vi "Digital_Bridge_3_kart.vi"() -> ()   [LabVIEW 2014] (continued)
                      n2699 = case shown="6" w6200 {
                        tunnel: [4.0 ("iterasyon WAGNER") w6203 w6204 w6205 w6206 w6207 w6208] -> w6199
                        frame 0, Default {
                        }
                        frame 1 {
                          n2700 = local read "Iterasyon Successful"() -> (w6203:dbl)
                        }
                        frame 2 {
                          n2701 = local read "Direnc 1 - Direnc 2"() -> (w6204:u32)
                        }
                        frame 3 {
                          n2702 = local read "olcum"() -> (w6205:u16)
                        }
                        frame 4 {
                          n2703 = local read "set"() -> (w6206:u16)
                        }
                        frame 5 {
                          n2704 = local read "frekans index"() -> (w6207:dbl)
                        }
                        frame 6 {
                          n2705 = local read "iterasyon WAGNER"() -> (w6208:dbl)
                        }
                      }
                      n2706 = Replace Array Subset(array=w6201, new element=w6199, index=w6200) -> (w6198:dbl[])
                    }
                    n2707 = local read "Output Denge Kosulu x2_y2"() -> (w6169:dbl[][])
                    n2708 = control-ref of="Default Values Listbox"() -> (w6148:refnum<vi>)
                    n2709 = local read "Output Denge Kosulu x1_x2"() -> (w6142:dbl[][])
                    n2710 = local read "Outpu Denge Kosulu y1_y2"() -> (w6143:dbl[][])
                    n2711 = local read "Cluster"() -> (w6146:T2)
                    n2712 = local read "Cluster 2"() -> (w6145:T1)
                    n2713 = local read "Frekanslar"() -> (w6129:dbl[])
                    n2714 = Array Size(array=w6129) -> (size(s)=w6128:i32)
                    n2715 = local read "default values"() -> (w6168:T3)
                    n2716 = local read "input values"() -> (w6147:dbl[])
                    n2717 = call "merge_x_y.vi"("frekans size"=w6128, "y1_y2"=w6143, "x1_x2"=w6142) -> ("x1_x2_y1_y2"=w6141:dbl[][])  [unwired: 8 in]
                    n2718 = local read "Sheet name"() -> (w6165:string)
                    n2719 = local read "Other Boolean Array"() -> (w6163:bool[])
                    n2720 = for {
                      N: 5 -> [_]
                      shift-right: [w6189] -> w6166
                      shift-left: w6163 -> [w6192]
                      i -> [w6191]
                      n2721 = case shown="0, Default" w6191 {
                        tunnel: [FALSE FALSE FALSE FALSE FALSE] -> w6190
                        frame 0, Default {
                        }
                        frame 1 {
                        }
                        frame 2 {
                        }
                        frame 3 {
                        }
                        frame 4 {
                        }
                      }
                      n2722 = Replace Array Subset(array=w6192, new element=w6190, index=w6191) -> (w6189:bool[])
                    }
                    n2723 = call "Pass.vi"("Other Array"=w6167, "Other Boolean Array"=w6166, "Denge Kosulu x2_y2"=w6169, "LstBox Refnum"=w6148, "Cluster"=w6146, "F/P Array Cluster"=w6145, "Sheet name"=w6165, "default values"=w6168, "x1_x2_y1_y2"=w6141, "input values"=w6147) -> ("output values"=w6140:dbl[], "Output Other Boolean Array"=w6161:bool[], "Output Cluster"=w6139:T2, "Output F/P Array Cluster"=w6135:T1, "output default values"=w6144:T11, "Output Iterasyon Successful"=w6162:dbl, "Denge Seçimi"=w6150:u8, "end time"=w6149:string)  [unwired: 1 in, 1 out]
                    n2724 = Unbundle By Name(w6139) -> ("F Values Array"=w6138:dbl[][], "control hz array"=w6137:dbl[][], "extra default values"=w6136:dbl[][])
                    n2725 = local write "input values"(w6140) -> ()
                    n2726 = Unbundle By Name(w6135) -> ("AD F/P Array"=w6134:dbl[][], "10R F/P Array"=w6133:dbl[][], "1R F/P Array"=w6132:dbl[][], "Wagner F/P Array"=w6131:dbl[][], "Kelvin F/P Array"=w6130:dbl[][])
                    n2727 = local write "default values"(w6144) -> ()
                    n2728 = local write "Iterasyon Successful"(w6162) -> ()
                    n2729 = local write "F Values Array"(w6138) -> ()
                    n2730 = local write "control hz array"(w6137) -> ()
                    n2731 = local write "extra default values"(w6136) -> ()
                    n2732 = local write "AD F/P Array"(w6134) -> ()
                    n2733 = local write "10R F/P Array"(w6133) -> ()
                    n2734 = local write "1R F/P Array"(w6132) -> ()
                    n2735 = local write "Wagner F/P Array"(w6131) -> ()
                    n2736 = local write "Kelvin F/P Array"(w6130) -> ()
                    n2737 = Index Array(array=w6161, index #1=0 ("index"), index #2=1 ("index"), index #3=2 ("index"), index #4=3 ("index"), index #5=4 ("index")) -> (element #1=w6155:bool, element #2=w6154:bool, element #3=w6153:bool, element #4=w6152:bool, element #5=w6151:bool)
                    n2738 = case shown="True" w6155 {
                      frame False {
                      }
                      frame True {
                        n2739 = local write "PASS WAGNER"(FALSE ("PASS WAGNER")) -> ()
                        n2740 = local write "reset values"(TRUE ("reset values")) -> ()
                        n2741 = local write "Boolean 4"(TRUE ("Boolean 4")) -> ()
                        n2742 = local write "pass hz"(TRUE ("pass hz")) -> ()
                      }
                    }
                    n2743 = case shown="True" w6154 {
                      tunnel: w6150 -> [_ w6183]
                      frame False {
                      }
                      frame True {
                        n2744 = local write "count meas"(u16 0 ("count meas")) -> ()
                        n2745 = local write "PASS WAGNER"(FALSE ("PASS WAGNER")) -> ()
                        n2746 = local write "Denge Seçimi"(w6183) -> ()
                        n2747 = local write "10R switch"(TRUE ("10R switch")) -> ()
                        n2748 = local write "Boolean 4"(TRUE ("Boolean 4")) -> ()
                      }
                    }
                    n2749 = case shown="True" w6153 {
                      tunnel: w6149 -> [_ w6178]
                      frame False {
                      }
                      frame True {
                        n2750 = local write "PASS WAGNER"(FALSE ("PASS WAGNER")) -> ()
                        n2751 = local write "reset values"(TRUE ("reset values")) -> ()
                        n2752 = local write "end time"(w6178) -> ()
                        n2753 = local write "Boolean 4"(TRUE ("Boolean 4")) -> ()
                      }
                    }
                    n2754 = case shown="True" w6152 {
                      frame False {
                      }
                      frame True {
                        n2755 = local write "PASS WAGNER"(FALSE ("PASS WAGNER")) -> ()
                        n2756 = local write "RESET SENS X 4"(TRUE ("RESET SENS X 4")) -> ()
                      }
                    }
                    n2757 = case shown="True" w6151 {
                      frame False {
                      }
                      frame True {
                        n2758 = local write "RESET SENS Y 4"(TRUE ("RESET SENS Y 4")) -> ()
                        n2759 = local write "PASS WAGNER"(FALSE ("PASS WAGNER")) -> ()
                      }
                    }
                  }
                  frame #3 {
                  }
                }
              }
            }
            n2760 = case shown="True" "auto phase wagner" {
              frame False {
              }
              frame True {
                n2761 = flat-sequence {
                  frame #0 {
                    n2762 = local read "GPIB In"() -> (w6293:refnum<visa-resource-name>)
                    n2763 = call "reference phase.vi"("Reference Phase (0.000 degrees)"="0", "VISA resource name"=w6293) -> ()  [unwired: 8 in, 2 out]
                  }
                  frame #1 {
                    w6295 = u16 0 items=["100 nV", "200 nV", "500 nV", "1 uV", "2 uV", "5 uV", "10 uV", "20 uV", "50 uV", "100 uV", "200 uV", "500 uV", "1 mV"] ("Min. Hassasiyet")
                    n2764 = local read "GPIB In"() -> (w6296:refnum<visa-resource-name>)
                    n2765 = local read "X Range W"() -> (w6294:dbl)
                    n2766 = call "GAIN BASIC.vi"("SR850 GPIB In"=w6296, "Max. Hassasiyet"=w6294, "Auto Gain (False)"=FALSE, "Min. Hassasiyet"=w6295) -> ()  [unwired: 10 in, 2 out]
                  }
                  frame #2 {
                    n2767 = local read "X 1.input W"() -> (w6298:dbl)
                    n2768 = global write "DB_Global_4_kart-Test.vi" "amplitude 1/1"(w6298) -> ()
                    n2769 = global write "DB_Global_4_kart-Test.vi" "phase 1/1"(w6298) -> ()
                  }
                  frame #3 {
                    n2770 = Wait (ms)(milliseconds to wait=u32 750) -> ()  [unwired: 1 out]
                  }
                  frame #4 {
                    n2771 = local write "auto phase wagner"(FALSE ("auto phase wagner")) -> ()
                    n2772 = local write "read x1 y1 4"(TRUE ("output x")) -> ()
                  }
                }
              }
            }
            n2773 = case shown="True" "read x1 y1 4" {
              frame False {
              }
              frame True {
                n2774 = local read "X Range W"() -> (w5999:dbl)
                n2775 = call "only_x_and_y_output.vi"("range"=w5999) -> ("cycle 2"=w5998:bool, "range 2"=w5995:dbl, "Output Y"=w5996:dbl, "Output X"=w5997:dbl)  [unwired: 7 in]
                n2776 = case shown="False" w5998 {
                  tunnel: w5997 -> [w6002 _]
                  tunnel: w5996 -> [w6001 _]
                  tunnel: w5995 -> [w6000 w6010]
                  frame False {
                    n2777 = flat-sequence {
                      tunnel: w6002 -> [w6005]
                      tunnel: w6001 -> [w6004]
                      tunnel: w6000 -> [w6003]
                      frame #0 {
                        n2778 = local write "X Range W"(w6003) -> ()
                        n2779 = local write "Output Y1"(w6004) -> ()
                        n2780 = local write "Output X1"(w6005) -> ()
                      }
                      frame #1 {
                        n2781 = local read "X 2.input W"() -> (w6006:dbl)
                        n2782 = global write "DB_Global_4_kart-Test.vi" "amplitude 1/1"(w6006) -> ()
                      }
                      frame #2 {
                        n2783 = Wait (ms)(milliseconds to wait=u32 750) -> ()  [unwired: 1 out]
                      }
                      frame #3 {
                        n2784 = local write "read x1 y1 4"(FALSE ("output x")) -> ()
                        n2785 = local write "read x2 y2 4"(TRUE ("output x")) -> ()
                      }
                    }
                  }
                  frame True {
                    n2786 = local write "X Range W"(w6010) -> ()
                  }
                }
              }
            }
            n2787 = case shown="True" "read x2 y2 4" {
              frame False {
              }
              frame True {
                n2788 = local read "X Range W"() -> (w5983:dbl)
                n2789 = call "only_x_and_y_output.vi"("range"=w5983) -> ("cycle 2"=w5982:bool, "range 2"=w5979:dbl, "Output Y"=w5980:dbl, "Output X"=w5981:dbl)  [unwired: 7 in]
                n2790 = case shown="False" w5982 {
                  tunnel: w5981 -> [w5986 _]
                  tunnel: w5980 -> [w5985 _]
                  tunnel: w5979 -> [w5984 w5994]
                  frame False {
                    n2791 = flat-sequence {
                      tunnel: w5986 -> [w5989]
                      tunnel: w5985 -> [w5988]
                      tunnel: w5984 -> [w5987]
                      frame #0 {
                        n2792 = local write "Output X2"(w5989) -> ()
                        n2793 = local write "Output Y2"(w5988) -> ()
                        n2794 = local write "X Range W"(w5987) -> ()
                      }
                      frame #1 {
                        n2795 = global write "DB_Global_4_kart-Test.vi" "amplitude 1/1"(0.0) -> ()
                      }
                      frame #2 {
                        n2796 = Wait (ms)(milliseconds to wait=u32 750) -> ()  [unwired: 1 out]
                      }
                      frame #3 {
                        n2797 = local write "result phase 4"(TRUE ("result phase 4")) -> ()
                        n2798 = local write "read x2 y2 4"(FALSE ("output y")) -> ()
                      }
                    }
                  }
                  frame True {
                    n2799 = local write "X Range W"(w5994) -> ()
                  }
                }
              }
            }
            n2800 = case shown="True" "RANGE KONTROL Y 4" {
              frame False {
              }
              frame True {
                n2801 = local read "Outpu Denge Kosulu y1_y2"() -> (w6086:dbl[][])
                n2802 = local read "iterasyon WAGNER"() -> (w6085:dbl)
                n2803 = local read "input 1 y [wagner]"() -> (w6087:dbl)
                n2804 = local read "input 2 y [wagner]"() -> (w6088:dbl)
                n2805 = local read "frekans index"() -> (w6079:dbl)
                n2806 = local read "output 2 y [wagner]"() -> (w6082:dbl)
                n2807 = local read "output 1 y [wagner]"() -> (w6084:dbl)
                n2808 = call "Range Kontrol Y.vi"("denge degeri"=4.0, "iterasyon Denge"=w6085, "frekans index"=w6079, "Denge Kosulu y1_y2"=w6086, "Yk"=w6087, "Y(k-1)"=w6088, "output y 1"=w6084, "output y 2"=w6082) -> ("Output Y(k-1)"=w6078:dbl, "result output y"=w6089:dbl, "KONTROL X"=w6081:bool, "IF ELSE"=w6080:bool)  [unwired: 8 in]
                n2809 = local write "Wagner Y(k-1)"(w6078) -> ()
                n2810 = local write "result output y [Wagner]"(w6089) -> ()
                n2811 = flat-sequence {
                  tunnel: w6081 -> [w6091]
                  tunnel: w6080 -> [w6090]
                  frame #0 {
                    n2812 = case shown="True" w6090 {
                      frame False {
                      }
                      frame True {
                        n2813 = local write "IF ELSE Y 4"(TRUE ("IF ELSE X 4")) -> ()
                      }
                    }
                    n2814 = case shown="True" w6091 {
                      frame False {
                      }
                      frame True {
                        n2815 = local write "KONTROL X 4"(TRUE ("KONTROL Y 4")) -> ()
                      }
                    }
                  }
                  frame #1 {
                    n2816 = local write "RANGE KONTROL Y 4"(FALSE ("KONTROL Y 4")) -> ()
                    n2817 = local read "İterasyon Y 4"() -> (w6094:dbl)
                    n2818 = Increment(x=w6094) -> (x+1=w6095:dbl)
                    n2819 = local write "İterasyon Y 4"(w6095) -> ()
                  }
                }
              }
            }
            n2820 = case shown="True" "Y 4" {
              frame False {
              }
              frame True {
                n2821 = local read "İterasyon Y 4"() -> (w6118:dbl)
                n2822 = local read "Wagner Y(k-1)"() -> (w6119:dbl)
                n2823 = call "Y.vi"("Y(k-1)"=w6119, "İterasyon Denge"=w6118, "denge degeri"=4.0) -> ("error"=w6116:bool, "output Y(k-1)"=w6113:dbl, "output y 1"=w6114:dbl, "cycle"=w6115:bool)  [unwired: 5 in]
                n2824 = case shown="False" w6115 {
                  tunnel: w6116 -> [w6122 _]
                  tunnel: w6114 -> [w6121 _]
                  tunnel: w6113 -> [w6120 _]
                  frame False {
                    n2825 = case shown="True" w6122 {
                      frame False {
                        n2826 = local write "Y 4"(FALSE ("X 4")) -> ()
                        n2827 = local write "Y1 4"(TRUE ("X1 4")) -> ()
                      }
                      frame True {
                        n2828 = local write "Y 4"(FALSE ("X 4")) -> ()
                        n2829 = local write "error"(TRUE ("X1 4")) -> ()
                      }
                    }
                    n2830 = local write "output 1 y [wagner]"(w6121) -> ()
                    n2831 = local write "Wagner Y(k-1)"(w6120) -> ()
                    n2832 = local write "input 2 y [wagner]"(w6120) -> ()
                  }
                  frame True {
                  }
                }
              }
            }
            n2833 = case shown="True" "RANGE KONTROL X 4" {
              frame False {
              }
              frame True {
                n2834 = local read "Output Denge Kosulu x1_x2"() -> (w6249:dbl[][])
                n2835 = local read "iterasyon WAGNER"() -> (w6251:dbl)
                n2836 = local read "input 1 x [wagner]"() -> (w6248:dbl)
                n2837 = local read "frekans index"() -> (w6250:dbl)
                n2838 = local read "input 2 x [wagner]"() -> (w6247:dbl)
                n2839 = local read "output 2 x [wagner]"() -> (w6246:dbl)
                n2840 = local read "output 1 x [wagner]"() -> (w6245:dbl)
                n2841 = call "Range Kontrol X.vi"("denge degeri"=4.0, "iterasyon Denge"=w6251, "frekans index"=w6250, "Denge Kosulu x1_x2"=w6249, "Xk"=w6248, "X(k-1)"=w6247, "output x 1"=w6245, "output x 2"=w6246) -> ("Output X(k-1)"=w6240:dbl, "result output x"=w6244:dbl, "KONTROL Y"=w6243:bool, "IF ELSE"=w6242:bool, "Start Denge Y"=w6241:bool)  [unwired: 7 in]
                n2842 = local write "Wagner  X(k-1)"(w6240) -> ()
                n2843 = local write "result output x [Wagner]"(w6244) -> ()
                n2844 = flat-sequence {
                  tunnel: w6243 -> [w6255]
                  tunnel: w6242 -> [w6254]
                  tunnel: w6241 -> [w6253]
                  frame #0 {
                    n2845 = case shown="True" w6253 {
                      frame False {
                      }
                      frame True {
                        n2846 = local write "Start Wagner Y"(TRUE ("Start Wagner Y")) -> ()
                      }
                    }
                    n2847 = case shown="True" w6254 {
                      frame False {
                      }
                      frame True {
                        n2848 = local write "IF ELSE X 4"(TRUE ("IF ELSE X 4")) -> ()
                      }
                    }
                    n2849 = case shown="True" w6255 {
                      frame False {
                      }
                      frame True {
                        n2850 = local write "KONTROL Y 4"(TRUE ("KONTROL Y 4")) -> ()
                      }
                    }
                  }
                  frame #1 {
                    n2851 = local write "RANGE KONTROL X 4"(FALSE ("KONTROL Y 4")) -> ()
                    n2852 = local read "İterasyon X 4"() -> (w6259:dbl)
                    n2853 = Increment(x=w6259) -> (x+1=w6260:dbl)
                    n2854 = local write "İterasyon X 4"(w6260) -> ()
                  }
                }
              }
            }
            n2855 = case shown="True" "X 4" {
              frame False {
              }
              frame True {
                n2856 = local read "Wagner  X(k-1)"() -> (w6284:dbl)
                n2857 = local read "İterasyon X 4"() -> (w6283:dbl)
                n2858 = call "X.vi"("X(k-1)"=w6284, "İterasyon Denge"=w6283, "denge degeri"=4.0) -> ("error"=w6280:bool, "output X(k-1)"=w6278:dbl, "output x 1"=w6279:dbl, "cycle"=w6281:bool)  [unwired: 5 in]
                n2859 = case shown="False" w6281 {
                  tunnel: w6280 -> [w6287 _]
                  tunnel: w6279 -> [w6286 _]
                  tunnel: w6278 -> [w6285 _]
                  frame False {
                    n2860 = case shown="True" w6287 {
                      frame False {
                        n2861 = local write "X 4"(FALSE ("X 4")) -> ()
                        n2862 = local write "X1 4"(TRUE ("X1 4")) -> ()
                      }
                      frame True {
                        n2863 = local write "error"(TRUE ("X1 4")) -> ()
                        n2864 = local write "X 4"(FALSE ("X 4")) -> ()
                      }
                    }
                    n2865 = local write "output 1 x [wagner]"(w6286) -> ()
                    n2866 = local write "Wagner  X(k-1)"(w6285) -> ()
                    n2867 = local write "input 2 x [wagner]"(w6285) -> ()
                  }
                  frame True {
                  }
                }
              }
            }
            n2868 = case shown="True" "result phase 4" {
              frame False {
              }
              frame True {
                n2869 = flat-sequence {
                  tunnel: [w5942] -> w5941
                  tunnel: w5941 -> [w5962]
                  tunnel: [w5962] -> w5940
                  tunnel: w5940 -> [w5967]
                  tunnel: [w5967] -> w5939
                  tunnel: w5939 -> [w5974]
                  frame #0 {
                    # "pi"
                    n2870 = local read "Output X2"() -> (w5947:dbl)
                    n2871 = local read "Output X1"() -> (w5948:dbl)
                    n2872 = local read "Output Y2"() -> (w5949:dbl)
                    n2873 = local read "Output Y1"() -> (w5950:dbl)
                    n2874 = local read "GPIB In"() -> (w5951:refnum<visa-resource-name>)
                    n2875 = call "return phase.vi"("VISA resource name"=w5951) -> ("return phase"=w5943:string)  [unwired: 10 in]
                    n2876 = Fract/Exp String To Number(use system decimal point (T)=FALSE, string=w5943) -> (number=w5945:dbl)  [unwired: 2 in, 1 out]
                    n2877 = formula code="theta = atan((y2-y1)/(x2-x1))*(180/pi)+phase;"("x1"=w5947, "x2"=w5948, "y1"=w5949, "y2"=w5950, "phase"=w5945, "pi"=3.141592653589793) -> ("theta"=w5942:dbl)
                  }
                  frame #1 {
                    n2878 = local read "frekans index"() -> (w5959:dbl)
                    n2879 = local read "Frekanslar"() -> (w5960:dbl[])
                    n2880 = local read "Cluster 2"() -> (w5954:T1)
                    n2881 = local read "Direnc 1 - Direnc 2"() -> (w5964:u32)
                    n2882 = property on="Default Values Listbox" class="LstBox (strict)"() -> ("Item Names"=w5961:string[])  [unwired: 2 in, 2 out]
                    n2883 = Fract/Exp String To Number(string=w5961) -> (number=w5958:dbl[])  [unwired: 3 in, 1 out]
                    n2884 = local read "Wagner F/P Array"() -> (w5965:dbl[][])
                    n2885 = Index Array(array=w5960, index=w5959) -> (element=w5956:dbl)
                    n2886 = Search 1D Array(1D array=w5958, element=w5956, start index (0)=0) -> (index of element=w5955:i32)
                    n2887 = Increment(x=w5964) -> (x+1=w5963:u32)
                    n2888 = Replace Array Subset(array=w5965, new element=w5962, index (row)=w5963, index (col)=w5955) -> (w5952:dbl[][])
                    n2889 = local write "Wagner F/P Array"(w5952) -> ()
                    n2890 = Bundle By Name(cluster=w5954, "Wagner F/P Array"=w5952) -> (w5953:T1)
                    n2891 = local write "Cluster 2"(w5953) -> ()
                  }
                  frame #2 {
                    n2892 = Wait (ms)(milliseconds to wait=u32 250) -> ()  [unwired: 1 out]
                  }
                  frame #3 {
                    w5971 = u16 0 items=["A", "A-B"] ("Input Source (0: A)")
                    n2893 = local read "GPIB In"() -> (w5970:refnum<visa-resource-name>)
                    n2894 = Number To Fractional String(number=w5974) -> (F-format string=w5968:string)  [unwired: 3 in]
                    n2895 = Search and Replace String(input string=w5968, search string=",", replace string="." ("replace string (\"\")")) -> (result string=w5969:string)  [unwired: 5 in, 3 out]
                    n2896 = call "reference phase.vi"("Reference Phase (0.000 degrees)"=w5969, "VISA resource name"=w5970) -> ("error out"=w5972:errorcluster, "VISA resource name out"=w5973:refnum<visa-resource-name>)  [unwired: 8 in]
                    n2897 = call "input source.vi"("error in (no error)"=w5972, "Input Source (0: A)"=w5971, "VISA resource name"=w5973) -> ()  [unwired: 7 in, 2 out]
                  }
                  frame #4 {
                    n2898 = local write "Contiune Wagner"(TRUE ("Contiune Wagner")) -> ()
                    n2899 = local write "result phase 4"(FALSE ("result phase 4")) -> ()
                  }
                }
              }
            }
            n2900 = case shown="True" "Y1 4" {
              frame False {
              }
              frame True {
                n2901 = local read "output 1 y [wagner]"() -> (w6105:dbl)
                n2902 = local read "İterasyon Y 4"() -> (w6102:dbl)
                n2903 = local read "Wagner Y(k-1)"() -> (w6104:dbl)
                n2904 = local read "Wagner Yk"() -> (w6103:dbl)
                n2905 = call "Y1.vi"("denge degeri"=4.0, "İterasyon Denge"=w6102, "Yk"=w6103, "Y(k-1)"=w6104, "output y 1"=w6105) -> ("Output Yk"=w6098:dbl, "output y 2"=w6097:dbl, "cycle"=w6099:bool, "error"=w6100:bool)  [unwired: 7 in]
                n2906 = case shown="False" w6099 {
                  tunnel: w6100 -> [w6108 _]
                  tunnel: w6098 -> [w6107 _]
                  tunnel: w6097 -> [w6106 _]
                  frame False {
                    n2907 = case shown="False" w6108 {
                      frame False {
                        n2908 = local write "RANGE KONTROL Y 4"(TRUE ("RANGE KONTROL X 4")) -> ()
                        n2909 = local write "Y1 4"(FALSE ("X1 4")) -> ()
                      }
                      frame True {
                        n2910 = local write "error"(TRUE ("RANGE KONTROL X 4")) -> ()
                        n2911 = local write "Y1 4"(FALSE ("X1 4")) -> ()
                      }
                    }
                    n2912 = local write "Wagner Yk"(w6107) -> ()
                    n2913 = local write "output 2 y [wagner]"(w6106) -> ()
                  }
                  frame True {
                  }
                }
              }
            }
            n2914 = case shown="True" "IF ELSE Y 4" {
              frame False {
              }
              frame True {
                n2915 = local read "input 1 y [wagner]"() -> (w6067:dbl)
                n2916 = local read "input 2 y [wagner]"() -> (w6068:dbl)
                n2917 = local read "output 1 y [wagner]"() -> (w6071:dbl)
                n2918 = local read "result output y [Wagner]"() -> (w6073:dbl)
                n2919 = local read "output 2 y [wagner]"() -> (w6072:dbl)
                n2920 = call "If Else Y.vi"("denge degeri"=4.0, "Yk"=w6067, "Y(k-1)"=w6068, "output y 1"=w6071, "output y 2"=w6072, "result output y"=w6073) -> ("Output Y(k-1)"=w6066:dbl, "Start Y"=w6069:bool)  [unwired: 8 in]
                n2921 = local write "Wagner Y(k-1)"(w6066) -> ()
                n2922 = case shown="True" w6069 {
                  frame False {
                  }
                  frame True {
                    n2923 = local read "count meas"() -> (w6075:u16)
                    n2924 = local write "RESET SENS Y 4"(TRUE ("START X 4")) -> ()
                    n2925 = local write "IF ELSE Y 4"(FALSE ("IF ELSE X 4")) -> ()
                    n2926 = Increment(x=w6075) -> (x+1=w6074:u16)
                    n2927 = local write "count meas"(w6074) -> ()
                  }
                }
              }
            }
            n2928 = case shown="True" "X1 4" {
              frame False {
              }
              frame True {
                n2929 = local read "output 1 x [wagner]"() -> (w6270:dbl)
                n2930 = local read "İterasyon X 4"() -> (w6267:dbl)
                n2931 = local read "Wagner  X(k-1)"() -> (w6269:dbl)
                n2932 = local read "Wagner Xk"() -> (w6268:dbl)
                n2933 = call "X1.vi"("denge degeri"=4.0, "İterasyon Denge"=w6267, "Xk"=w6268, "X(k-1)"=w6269, "output x 1"=w6270) -> ("Output Xk"=w6263:dbl, "output x 2"=w6262:dbl, "cycle"=w6264:bool, "error"=w6265:bool)  [unwired: 7 in]
                n2934 = case shown="False" w6264 {
                  tunnel: w6265 -> [w6273 _]
                  tunnel: w6263 -> [w6272 _]
                  tunnel: w6262 -> [w6271 _]
                  frame False {
                    n2935 = case shown="True" w6273 {
                      frame False {
                        n2936 = local write "RANGE KONTROL X 4"(TRUE ("RANGE KONTROL X 4")) -> ()
                        n2937 = local write "X1 4"(FALSE ("X1 4")) -> ()
                      }
                      frame True {
                        n2938 = local write "error"(TRUE ("RANGE KONTROL X 4")) -> ()
                        n2939 = local write "X1 4"(FALSE ("X1 4")) -> ()
                      }
                    }
                    n2940 = local write "Wagner Xk"(w6272) -> ()
                    n2941 = local write "output 2 x [wagner]"(w6271) -> ()
                  }
                  frame True {
                  }
                }
              }
            }
            n2942 = case shown="True" "IF ELSE X 4" {
              frame False {
              }
              frame True {
                n2943 = local read "input 1 x [wagner]"() -> (w6229:dbl)
                n2944 = local read "input 2 x [wagner]"() -> (w6230:dbl)
                n2945 = local read "result output x [Wagner]"() -> (w6235:dbl)
                n2946 = local read "output 1 x [wagner]"() -> (w6233:dbl)
                n2947 = local read "output 2 x [wagner]"() -> (w6234:dbl)
                n2948 = call "If Else X.vi"("denge degeri"=4.0, "Xk"=w6229, "X(k-1)"=w6230, "output x 1"=w6233, "output x 2"=w6234, "result output x"=w6235) -> ("Output X(k-1)"=w6228:dbl, "Start X"=w6231:bool)  [unwired: 8 in]
                n2949 = local write "Wagner  X(k-1)"(w6228) -> ()
                n2950 = case shown="True" w6231 {
                  frame False {
                  }
                  frame True {
                    n2951 = local read "count meas"() -> (w6236:u16)
                    n2952 = local write "RESET SENS X 4"(TRUE ("START X 4")) -> ()
                    n2953 = local write "IF ELSE X 4"(FALSE ("IF ELSE X 4")) -> ()
                    n2954 = Increment(x=w6236) -> (x+1=w6237:u16)
                    n2955 = local write "count meas"(w6237) -> ()
                  }
                }
              }
            }
            n2956 = case shown="True" "KONTROL X 4" {
              frame False {
              }
              frame True {
                n2957 = local read "Output Denge Kosulu x1_x2"() -> (w6055:dbl[][])
                n2958 = local read "iterasyon WAGNER"() -> (w6047:dbl)
                n2959 = local read "Manuel/Otomatik"() -> (w6054:enum16{"Manuel", "Otomatik"})
                n2960 = local read "frekans index"() -> (w6048:dbl)
                n2961 = call "Kontrol X.vi"("denge degeri"=4.0, "İterasyon Denge"=w6047, "Denge Kosulu x1_x2"=w6055, "Manuel/Otomatik"=w6054, "frekans index"=w6048) -> ("Denge Seçimi"=w6051:u8, "New İterasyon Denge"=w6050:dbl, "Iterasyon Count Successful"=w6049:dbl, "Start Denge X"=w6052:bool)  [unwired: 7 in]
                n2962 = case shown="True" w6052 {
                  tunnel: w6051 -> [w6063 _]
                  tunnel: w6050 -> [_ _]
                  tunnel: w6049 -> [w6062 _]
                  frame False {
                    n2963 = local write "Iterasyon Successful"(w6062) -> ()
                    n2964 = local write "10R switch"(TRUE ("10R switch")) -> ()
                    n2965 = local write "Denge Seçimi"(w6063) -> ()
                    n2966 = local read "iterasyon WAGNER"() -> (w6057:dbl)
                    n2967 = local write "count meas"(u16 0 ("count meas")) -> ()
                    n2968 = local write "KONTROL X 4"(FALSE ("KONTROL X 4")) -> ()
                    n2969 = local write "Boolean 4"(TRUE ("Boolean 4")) -> ()
                    n2970 = Increment(x=w6057) -> (x+1=w6056:dbl)
                    n2971 = local write "iterasyon WAGNER"(w6056) -> ()
                  }
                  frame True {
                    n2972 = local write "RESET SENS X 4"(TRUE ("Start Wagner Y")) -> ()
                    n2973 = local write "KONTROL X 4"(FALSE ("KONTROL X 4")) -> ()
                  }
                }
              }
            }
            n2974 = case shown="True" "KONTROL Y 4" {
              frame False {
              }
              frame True {
                n2975 = local read "Outpu Denge Kosulu y1_y2"() -> (w6217:dbl[][])
                n2976 = local read "iterasyon WAGNER"() -> (w6209:dbl)
                n2977 = local read "Manuel/Otomatik"() -> (w6216:enum16{"Manuel", "Otomatik"})
                n2978 = local read "frekans index"() -> (w6210:dbl)
                n2979 = call "Kontrol Y.vi"("denge degeri"=4.0, "İterasyon Denge"=w6209, "Denge Kosulu y1_y2"=w6217, "Manuel/Otomatik"=w6216, "frekans index"=w6210) -> ("Denge Seçimi"=w6213:u8, "New İterasyon Denge"=w6212:dbl, "Iterasyon Count Successful"=w6211:dbl, "Start Denge Y"=w6214:bool)  [unwired: 7 in]
                n2980 = case shown="True" w6214 {
                  tunnel: w6213 -> [w6225 _]
                  tunnel: w6212 -> [_ _]
                  tunnel: w6211 -> [w6224 _]
                  frame False {
                    n2981 = local write "Iterasyon Successful"(w6224) -> ()
                    n2982 = local write "10R switch"(TRUE ("10R switch")) -> ()
                    n2983 = local write "Denge Seçimi"(w6225) -> ()
                    n2984 = local read "iterasyon WAGNER"() -> (w6219:dbl)
                    n2985 = local write "count meas"(u16 0 ("count meas")) -> ()
                    n2986 = local write "KONTROL Y 4"(FALSE ("KONTROL Y 4")) -> ()
                    n2987 = local write "Boolean 4"(TRUE ("Boolean 4")) -> ()
                    n2988 = Increment(x=w6219) -> (x+1=w6218:dbl)
                    n2989 = local write "iterasyon WAGNER"(w6218) -> ()
                  }
                  frame True {
                    n2990 = local write "KONTROL Y 4"(FALSE ("KONTROL Y 4")) -> ()
                    n2991 = local write "RESET SENS Y 4"(TRUE ("Start Wagner Y")) -> ()
                  }
                }
              }
            }
          }
          frame 5 {
            # "Bu bölümde, ilgili denge durumunun dengede olup olmadığı kontrol edilir.\n\nEğer denge sağlanmışsa, program doğrudan bir sonraki denge aşamasına geçer.\n\nAyrıca, tüm dengeler başarıyla tamamlanmış ve belirlenen ölçüm sayısına ulaşılmışsa, veriler bu alt program (subVI) aracılığıyla Excel dosyasına aktarılır."
            # "Bu bölümde, Y değerinin dengelendiği kabul edilerek, şimdi sıra X değerinin dengede olup olmadığını kontrol etmeye gelir. \n\nEğer X de dengedeyse, program bir sonraki işlem için ilgili switch case’i aktif eder. \n\nAncak Y dengede değilse, program X’i dengelemeye yönelik işlemlere yönlendirilir."
            # "Bu bölümde, X değerinin dengelendiği kabul edilerek, şimdi sıra Y değerinin dengede olup olmadığını kontrol etmeye gelir. \n\nEğer Y de dengedeyse, program bir sonraki işlem için ilgili switch case’i aktif eder. \n\nAncak Y dengede değilse, program Y’yi dengelemeye yönelik işlemlere yönlendirilir."
            # "IF ELSE X 5 ile benzer görevi üstleniyor sadece değerler Y oluyor"
            # "Range Kontrol X 5 ile benzer görevi üstleniyor sadece değerler Y oluyor"
            # "X1 5 ile benzer görevi üstleniyor sadece değerler Y oluyor"
            # "X 5 ile benzer görevi üstleniyor sadece değerler Y oluyor"
            # "Bu bölümün temel amacı, ölçüm aralığını (range) artırmaktır. Program, cihazdan gelen X ve Y değerlerini okuyarak bu değerlerin belirlenen aralık içinde olup olmadığını kontrol eder. \n\nEğer değerler aralık dışındaysa, aralık tekrar artırılır ve ölçüm yeniden yapılır. \n\nAyrıca, bu süreçte input ve output değerleri global değişkenlere kaydedilir. Çünkü sonraki turda, bu kaydedilen değerler farklı bir ölçüm aralığında eğim hesaplaması için kullanılacaktır."
            # "Bu bölümde, sıfırlanacak değer cihazdan okunur. Eğer okunan değer denge koşulunu sağlıyorsa, program Kontrol Y Case’ine geçer. \n\nAncak denge koşulu sağlanmazsa, program if-else yapısına yönlendirilir ve buna göre işlem devam eder."
            # "Bu bölümde, cihaza ikinci input değeri uygulanır ve karşılık gelen output değeri okunur. Daha sonra, hem input hem de output değerleri bir formüle yerleştirilir. Bu formül sayesinde, cihazın 0’a eşitleyeceği (sıfırlayacağı) yeni bir input değeri hesaplanır ve bu değer cihaza uygulanır."
            # "Bu bölümde ilk olarak giriş (input) değeri sisteme uygulanır. Eğer program ilk kez çalıştırılıyorsa, global input üzerinden belirlenen ilk değer (genellikle 0 V) kullanılır. \n\nArdından, cihazdan X değerleri okunur. Bu işlem 10 kez tekrarlanır ve elde edilen ölçümlerin ortalaması alınarak bir sonuç değeri elde edilir. Bu ortalama değer, daha sonra yapılacak işlemlerde kullanılmak üzere saklanır. Özellikle, formül içinde X değerini sıfırlamak için bu bilgiye ihtiyaç duyulur. \n\nEğer girilen input değeri 8 V’tan büyükse, bu durum sistem için güvenli olmayabileceğinden program hata (error) verir ve işlemi durdurur."
            # "Auto Phase, Read X1 Y1, Read X2 Y2, Result Phase: \n\nBu bölümler genel olarak faz ölçümü işlemini gerçekleştirir. \n\nİlk olarak, faz değeri 0’a sıfırlanır. Ardından, global input üzerinden belirlenen range (ölçüm aralığı) değeri uygulanır. Bu işlemden sonra yine global input’ta tanımlanmış olan: \n\nInput 1 verilir ve okuma yapılır (Read X1 Y1) \n\nInput 2 verilir ve okuma yapılır (Read X2 Y2) \n\nBu iki ölçüm sonucuna göre faz değeri bir formül yardımıyla hesaplanır. Elde edilen bu yeni faz değeri, ilgili F/P (frekans/faz) dizisine aktarılır. \n\nBu işlemler, sistemin doğru fazla çalışmasını sağlamak ve sonraki işlemlerde bu bilgiyi referans olarak kullanmak için gerçekleştirilir."
            # "Start X 5 ile benzer görevi üstleniyor sadece değerler Y oluyor"
            # "Reset Sens X 5 ile benzer görevi üstleniyor sadece değerler Y oluyor"
            # "Start Kelvin X ile benzer görevi üstleniyor sadece değerler Y oluyor"
            # "Pass subvi girmeden önce doğru range miyiz değil miyiz ölçüyor, değil ise +2 üst kademeye gidiyor"
            # "Bu bölümde, ölçüm için gerekli olan giriş (input) değerleri sisteme girilir. Girişler tamamlandıktan sonra program, ölçüm işlemini başlatmak üzere X adlı bölüme yönlendirilir. Bu adım, ölçüm sürecinin fiilen başlatıldığı ilk noktadır."
            # "Bu bölümde öncelikle, sistemin kaç kez ölçüm yaptığına işaret eden meas number (ölçüm sayısı) kontrol edilir. \nEğer bu sayı 6’dan büyükse (bu sınır kullanıcı tarafından belirlenmiştir ve değiştirilebilir), program hata verir ve reset values adlı bölüme yönlenir. Bu durum, sistemin çok fazla başarısız deneme yapmasını engellemek içindir. \nEğer ölçüm sayısı 6’dan küçükse, program global bir değişken olan sensitivity (duyarlılık) değerini ayarlar ve ardından işlemlere devam etmek üzere Start X bölümüne geçer."
            # "Bu bölümde, daha önce iterasyon (tekrarlama) yapılıp yapılmadığına bakılarak, programın hangi yöne devam edeceğine karar verilir. \n\nEğer gerekli ise, range kontrolü (ölçüm aralığının uygunluğu) yapılır veya sensitivity ayarlama (cihazın duyarlılığını belirleme) bölümlerine yönlendirilir. Bu sayede sistem, ölçüm koşullarına en uygun şekilde ayarlanarak doğru ve güvenilir sonuçlar elde edilmesi sağlanır."
            # "Bu bölümde, daha önce belirlenen F/P dizilerindeki (frekans/faz değerleri) faz bilgileri, mevcut frekansa göre uygulanır. Ardından, ilgili denge koşulunun daha önce gerçekleştirilip gerçekleştirilmediği kontrol edilir. \nEğer bu denge daha önce sağlanmamışsa, program uygun faz ayarlamasını yapar. Ancak denge daha önce zaten kurulmuşsa, faz ayarı yapılmadan işleme devam edilir. Bu sayede gereksiz tekrarların önüne geçilmiş olur."
            # "Bu bölüm, iterasyona (tekrarlamalı işleme) bağlı olarak Reserve ayarının maksimumda mı yoksa minimumda mı olacağını belirler. Aynı zamanda, ölçüm sürecinin başlangıcında kullanılacak olan sensitivity  değerleri de bu bölümde ayarlanır. Bu ayarlar, ölçüm sırasında cihazın hassasiyetini ve çalışma aralığını doğru şekilde belirlemek için gereklidir."
            # "kelvin"
            n2992 = case shown="True" "Start Kelvin X" {
              frame False {
              }
              frame True {
                n2993 = flat-sequence {
                  frame #0 {
                    w6842 = u16 1 items=["A", "A-B"] ("Input Source (0: A)")
                    n2994 = local read "frekans index"() -> (w6837:dbl)
                    n2995 = local read "Frekanslar"() -> (w6838:dbl[])
                    n2996 = local read "Direnc 1 - Direnc 2"() -> (w6839:u32)
                    n2997 = local read "Kelvin F/P Array"() -> (w6840:dbl[][])
                    n2998 = Index Array(array=w6838, index=w6837) -> (element=w6836:dbl)
                    n2999 = call "get_phase_element.vi"("index r"=w6839, "hz"=w6836, "Array"=w6840) -> ("element"=w6832:dbl)  [unwired: 8 in]
                    n3000 = Number To Fractional String(number=w6832) -> (F-format string=w6835:string)  [unwired: 3 in]
                    n3001 = local read "GPIB In"() -> (w6841:refnum<visa-resource-name>)
                    n3002 = Search and Replace String(input string=w6835, search string=",", replace string="." ("replace string (\"\")")) -> (result string=w6831:string)  [unwired: 5 in, 3 out]
                    n3003 = call "reference phase.vi"("Reference Phase (0.000 degrees)"=w6831, "VISA resource name"=w6841) -> ("error out"=w6843:errorcluster, "VISA resource name out"=w6844:refnum<visa-resource-name>)  [unwired: 8 in]
                    n3004 = call "input source.vi"("error in (no error)"=w6843, "Input Source (0: A)"=w6842, "VISA resource name"=w6844) -> ()  [unwired: 7 in, 2 out]
                  }
                  frame #1 {
                    n3005 = local read "İterasyon X 5"() -> (w6859:dbl)
                    n3006 = local read "1 or 10"() -> (w6858:i32)
                    n3007 = local read "frekans index"() -> (w6854:dbl)
                    n3008 = local read "control hz array"() -> (w6850:dbl[][])
                    n3009 = Greater?(x=w6859, y=0.0) -> (0:w6855:bool)
                    n3010 = call "change2d.vi"("reset(default false)"=FALSE, "index (col)"=w6854, "index (row)"=2, "read/write(T/F)"=TRUE, "2D Array"=w6850) -> ("result count"=w6849:dbl)  [unwired: 5 in, 1 out]
                    n3011 = Equal?(x=w6858, y=1) -> (x = y?=w6856:bool)
                    n3012 = local read "set"() -> (w6848:u16)
                    n3013 = Or(x=w6855, y=w6856) -> (x .or. y?=w6846:bool)
                    n3014 = Equal?(x=w6849, y=w6848) -> (x = y?=w6847:bool)
                    n3015 = Or(x=w6846, y=w6847) -> (x .or. y?=w6845:bool)
                    n3016 = case shown="True" w6845 {
                      frame False {
                        n3017 = local write "auto phase kelvin"(TRUE ("auto phase 10R")) -> ()
                        n3018 = local write "Start Kelvin X"(FALSE ("auto phase 10R")) -> ()
                      }
                      frame True {
                        n3019 = local write "Contiune Kelvin"(TRUE) -> ()
                        n3020 = local write "Start Kelvin X"(FALSE ("START WAGNER")) -> ()
                      }
                    }
                  }
                }
              }
            }
            n3021 = case shown="True" "Start Kelvin Y" {
              frame False {
              }
              frame True {
                n3022 = flat-sequence {
                  frame #0 {
                    w6939 = u16 1 items=["A", "A-B"] ("Input Source (0: A)")
                    n3023 = local read "frekans index"() -> (w6933:dbl)
                    n3024 = local read "Frekanslar"() -> (w6934:dbl[])
                    n3025 = local read "Direnc 1 - Direnc 2"() -> (w6936:u32)
                    n3026 = local read "Kelvin F/P Array"() -> (w6937:dbl[][])
                    n3027 = Index Array(array=w6934, index=w6933) -> (element=w6935:dbl)
                    n3028 = call "get_phase_element.vi"("index r"=w6936, "hz"=w6935, "Array"=w6937) -> ("element"=w6929:dbl)  [unwired: 8 in]
                    n3029 = Number To Fractional String(number=w6929) -> (F-format string=w6930:string)  [unwired: 3 in]
                    n3030 = Search and Replace String(input string=w6930, search string=",", replace string="." ("replace string (\"\")")) -> (result string=w6928:string)  [unwired: 5 in, 3 out]
                    n3031 = local read "GPIB In"() -> (w6938:refnum<visa-resource-name>)
                    n3032 = call "reference phase.vi"("Reference Phase (0.000 degrees)"=w6928, "VISA resource name"=w6938) -> ("error out"=w6940:errorcluster, "VISA resource name out"=w6941:refnum<visa-resource-name>)  [unwired: 8 in]
                    n3033 = call "input source.vi"("error in (no error)"=w6940, "Input Source (0: A)"=w6939, "VISA resource name"=w6941) -> ()  [unwired: 7 in, 2 out]
                  }
                  frame #1 {
                    n3034 = local write "Start Kelvin Y"(FALSE ("START Y 6")) -> ()
                    n3035 = local write "Boolean 5"(FALSE ("Boolean 4")) -> ()
                    n3036 = local write "RESET SENS Y 5"(TRUE ("START X")) -> ()
                  }
                }
              }
            }
            n3037 = case shown="True" "RESET SENS Y 5" {
              frame False {
              }
              frame True {
                n3038 = local read "iterasyon KELVIN"() -> (w6907:dbl)
                n3039 = local read "count meas"() -> (w6908:u16)
                n3040 = Greater?(x=w6908, y=u16 8) -> (0:w6905:bool)
                n3041 = Greater?(x=w6907, y=5.0) -> (0:w6904:bool)
                n3042 = Or(x=w6905, y=w6904) -> (x .or. y?=w6903:bool)
                n3043 = case shown="True" w6903 {
                  frame False {
                    n3044 = flat-sequence {
                      frame #0 {
                        n3045 = global read "show_sensitivity.vi" "show sensitivity (kelvin  y)"() -> (w6910:dbl)
                        n3046 = local read "GPIB In"() -> (w6911:refnum<visa-resource-name>)
                        n3047 = call "get_sensitivity.vi"("input 1"=w6910, "SR850 GPIB In"=w6911) -> ()  [unwired: 8 in, 2 out]
                      }
                      frame #1 {
                        n3048 = Wait (ms)(milliseconds to wait=u32 500) -> ()  [unwired: 1 out]
                      }
                      frame #2 {
                        n3049 = local write "RESET SENS Y 5"(FALSE ("RESET SENS X")) -> ()
                        n3050 = local write "START Y 5"(TRUE ("START X 4")) -> ()
                      }
                    }
                  }
                  frame True {
                    n3051 = local read "iterasyon KELVIN"() -> (w6916:dbl)
                    n3052 = Greater?(x=w6916, y=5.0) -> (0:w6915:bool)
                    n3053 = case shown="False" w6915 {
                      frame False {
                        n3054 = flat-sequence {
                          frame #0 {
                            n3055 = local write "count meas"(u16 9 ("count meas")) -> ()
                            n3056 = local write "İterasyon X 5"(0.0 ("İterasyon X 5")) -> ()
                            n3057 = local write "RESET SENS Y 5"(FALSE ("Start 10R X")) -> ()
                          }
                          frame #1 {
                            n3058 = local write "reset values"(TRUE ("Start 10R X")) -> ()
                            n3059 = local write "error"(TRUE ("Start 10R X")) -> ()
                          }
                        }
                      }
                      frame True {
                        n3060 = flat-sequence {
                          frame #0 {
                            n3061 = local write "count meas"(u16 10 ("count meas")) -> ()
                            n3062 = local write "İterasyon X 5"(0.0 ("İterasyon X 5")) -> ()
                            n3063 = local write "RESET SENS Y 5"(FALSE ("Start 10R X")) -> ()
                          }
                          frame #1 {
                            n3064 = local write "reset values"(TRUE ("Start 10R X")) -> ()
                            n3065 = local write "error"(TRUE ("Start 10R X")) -> ()
                          }
                        }
                      }
                    }
                  }
                }
              }
            }
            n3066 = case shown="True" "START Y 5" {
              frame False {
              }
              frame True {
                n3067 = flat-sequence {
                  frame #0 {
                    n3068 = local read "Kelvin Y(k-1)"() -> (w6946:dbl)
                    n3069 = local read "Kelvin Yk"() -> (w6945:dbl)
                    n3070 = local write "input 1 y [kelvin]"(w6945) -> ()
                    n3071 = local write "input 2 y [kelvin]"(w6946) -> ()
                    n3072 = global write "DB_Global_4_kart-Test.vi" "phase 2/1"(w6945) -> ()
                  }
                  frame #1 {
                    n3073 = Wait (ms)(milliseconds to wait=u32 500) -> ()  [unwired: 1 out]
                  }
                  frame #2 {
                    n3074 = local write "START Y 5"(FALSE ("START X")) -> ()
                    n3075 = local write "Y 5"(TRUE ("START X")) -> ()
                  }
                }
              }
            }
            n3076 = case shown="True" "kelvin switch" {
              frame False {
              }
              frame True {
                n3077 = flat-sequence {
                  frame #0 {
                    n3078 = local read "iterasyon KELVIN"() -> (w6865:dbl)
                    n3079 = Equal?(x=w6865, y=0.0) -> (x = y?=w6866:bool)
                    n3080 = case shown="True" w6866 {
                      frame False {
                      }
                      frame True {
                        n3081 = local read "1 or 10"() -> (w6868:i32)
                        n3082 = case shown="1" w6868 {
                          frame 0, Default {
                          }
                          frame 1 {
                            n3083 = local write "iterasyon KELVIN"(1.0 ("iterasyon WAGNER")) -> ()
                          }
                        }
                      }
                    }
                  }
                  frame #1 {
                    n3084 = local read "iterasyon KELVIN"() -> (w6875:dbl)
                    n3085 = local read "1 or 10"() -> (w6873:i32)
                    n3086 = Equal?(x=w6873, y=1) -> (x = y?=w6874:bool)
                    n3087 = Greater?(x=w6875, y=0.0) -> (0:w6871:bool)
                    n3088 = Or(x=w6871, y=w6874) -> (x .or. y?=w6870:bool)
                    n3089 = case shown="True" w6870 {
                      frame False {
                        n3090 = local read "Reserve Kelvin"() -> (w6878:u16)
                        n3091 = case shown="0, Default" w6878 {
                          tunnel: ["0" ("Reserve(MAX-MIN)") "1" ("Reserve(MAX-MIN)") "2" ("Reserve(MAX-MIN)")] -> w6877
                          frame 0, Default {
                          }
                          frame 1 {
                          }
                          frame 2 {
                          }
                        }
                        n3092 = local read "GPIB In"() -> (w6879:refnum<visa-resource-name>)
                        n3093 = call "Reserve.vi"("Reserve(MAX-MIN)"=w6877, "VISA resource name"=w6879) -> ()  [unwired: 8 in, 2 out]
                      }
                      frame True {
                        n3094 = local read "GPIB In"() -> (w6884:refnum<visa-resource-name>)
                        n3095 = call "Reserve.vi"("Reserve(MAX-MIN)"="2", "VISA resource name"=w6884) -> ()  [unwired: 8 in, 2 out]
                      }
                    }
                  }
                  frame #2 {
                    n3096 = Wait (ms)(milliseconds to wait=u32 500) -> ()  [unwired: 1 out]
                  }
                  frame #3 {
                    w6887 = u16 1 items=["Wagner", "Ground"] ("Switch")
                    w6888 = u16 1 items=["Open All", "Ana Denge", "10R", "1R"] ("Ring")
                    n3097 = call "mux1.vi"("Ring"=w6888) -> ("error out"=w6889:errorcluster)  [unwired: 9 in]
                    n3098 = property on="Tab Control" class="TabCtl (strict)"("Value"=T4."Kelvin" ("Tab Control")) -> ()  [unwired: 2 in, 2 out]
                    n3099 = call "mux2.vi"("Switch"=w6887, "error in (no error)"=w6889) -> ()  [unwired: 6 in, 1 out]
                  }
                  frame #4 {
                    n3100 = Wait (ms)(milliseconds to wait=u32 1000) -> ()  [unwired: 1 out]
                  }
                  frame #5 {
                    n3101 = local read "İterasyon X 5"() -> (w6897:dbl)
                    n3102 = local read "1 or 10"() -> (w6894:i32)
                    n3103 = Equal?(x=w6894, y=1) -> (x = y?=w6893:bool)
                    n3104 = Greater?(x=w6897, y=0.0) -> (0:w6892:bool)
                    n3105 = Or(x=w6892, y=w6893) -> (x .or. y?=w6891:bool)
                    n3106 = case shown="False" w6891 {
